vi "ConfigFunction.vi"(8 "error in (no error)":errorcluster, 11 "IviFgen in":refnum<class "IviFgen.lvclass">) -> (0 "error out":errorcluster, 3 "IviFgen out":refnum<class "IviFgen.lvclass">)   [LabVIEW 2014, in "FgenPlugins.lvlib" / "IviFgen.lvclass"]
uses:
  IviFgen.lvclass
  FgenPluginBaseClass/FgenPluginsBase.lvclass/FgenPluginsBase.ctl
  MemberClasses/StandardFunction/TypeDefs/StdWfrms.ctl
  MemberClasses/StandardFunction/TypeDefs/StdWfrm.ctl
  MemberClasses/ArbitraryFunction/TypeDefs/Arbitrary.ctl
  FgenPluginBaseClass/Accessors/Read Channels.vi
  FgenPluginBaseClass/Accessors/Read Mode (Function).vi
  FgenPluginBaseClass/Accessors/Read FunctionClass.vi
  MemberClasses/FunctionBaseClass/FunctionBase.lvclass
  MemberClasses/StandardFunction/StandardFunction.lvclass
  MemberClasses/ArbitraryFunction/ArbitraryFunction.lvclass
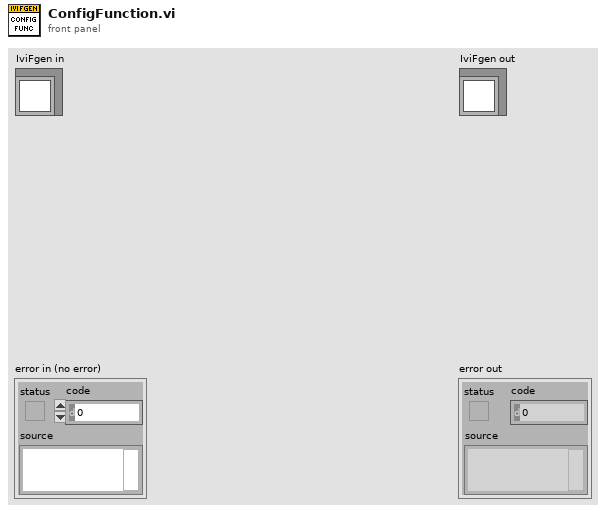
[diagram p1: front panel]
types:
  T1 = typedef "Functions.lvlib/StandardFunction.lvclass/StdWfrms.ctl" = cluster{"Count":u16, "StandardWfrm":T2[]}
  T2 = typedef "Functions.lvlib/StandardFunction.lvclass/StdWfrm.ctl" = cluster{"Amplitude":dbl, "DcOffset":dbl, "DutyCycle":dbl, "Frequency":dbl, "Phase":dbl, "Waveform":enum16{"Sine", "Square", "Triangle", "Ramp Up", "Ramp Down", "DC"}, "Handle":string}
  T3 = typedef "Functions.lvlib/ArbitraryFunction.lvclass/Arbitrary.ctl" = cluster{"Handle":string, "Size":i32, "Gain":dbl, "Offset":dbl, "Waveform":waveform(dbl)}
  T4 = typedef "FgenPlugins.lvlib/Channel.ctl" = cluster{"Name":string, "Enabled":bool, "Operation":enum16{"Continuous", "Burst"}, "Impedance (50)":dbl, "Handle":string, "Connected":bool, "Mode (Function)":enum16{"Function", "Arbitrary", "Sequence"}}
  T5 = enum16{"Sine", "Square", "Triangle", "Ramp Up", "Ramp Down", "DC"}
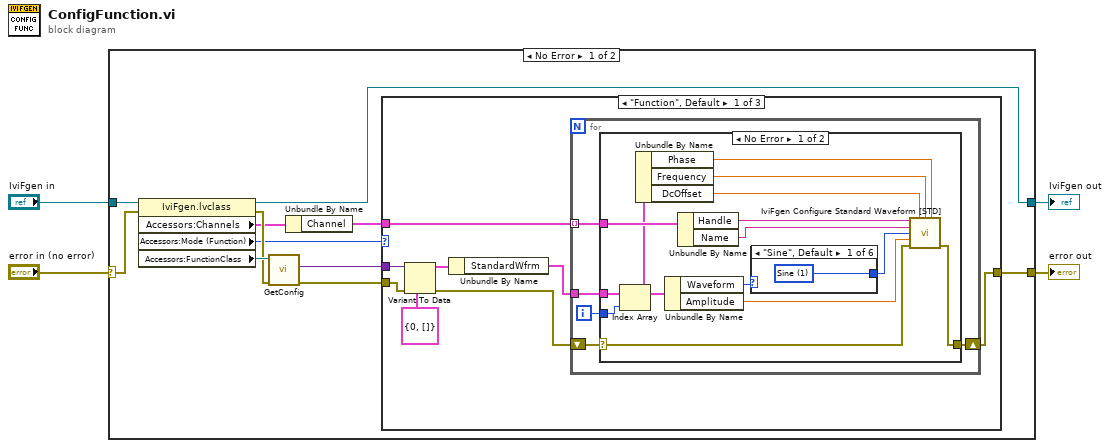
[diagram p0: block diagram]
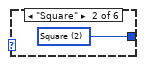
[diagram p2: hidden frame]
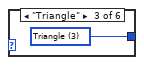
[diagram p3: hidden frame]
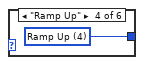
[diagram p4: hidden frame]
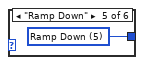
[diagram p5: hidden frame]
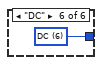
[diagram p6: hidden frame]
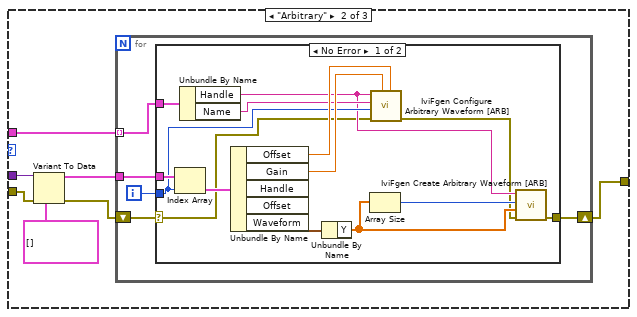
[diagram p8: hidden frame]
diagram:
  n1 = case shown="No Error" "error in (no error)" {
    selector: "error in (no error)" -> [w14 w79]
    tunnel: "IviFgen in" -> [w15 w78]
    tunnel: [w9 w79] -> w2
    tunnel: [w5 w78] -> w1
    frame No Error {
      n2 = property class="IviFgen.lvclass"(reference=w15, error in=w14) -> (reference out=w5:refnum<class "IviFgen.lvclass">, error out=w11:errorcluster, "Accessors:Channels"=w7:cluster{"Count":u16, "Channel":T4[]}, "Accessors:Mode (Function)"=w8:enum16{"Function", "Arbitrary", "Sequence"}, "Accessors:FunctionClass"=w13:refnum<class "FunctionBase.lvclass">)
      n3 = call-dynamic "GetConfig.vi"("error in (no error)"=w11, "FunctionBase in"=w13) -> ("error out"=w10:errorcluster, "Config"=w12:variant)  [unwired: 7 in, 1 out]
      n4 = Unbundle By Name(w7) -> ("Channel"=w6:T4[])
      n5 = case shown="\"Function\", Default" w8 {
        tunnel: w12 -> [w22 w56 _]
        tunnel: w10 -> [w23 w55 w77]
        tunnel: [w17 w50 w77] -> w9
        tunnel: w6 -> [w16 w53 _]
        frame "Function", Default {
          n6 = Variant To Data(error in=w23, type=T1 {"Count"=0, "StandardWfrm"=[]} ("StandardWfrms"), Variant=w22) -> (data=w20:T1, error out=w18:errorcluster)
          n7 = Unbundle By Name(w20) -> ("StandardWfrm"=w19:T2[])
          n8 = for {
            tunnel: w16 -> [w26] mode=indexing
            tunnel: w19 -> [w28]
            shift-right: [w24] -> w17
            shift-left: w18 -> [w25]
            i -> [w27]
            n9 = case shown="No Error" w25 {
              selector: w25 -> [w32 w49]
              tunnel: w28 -> [w42 _]
              tunnel: w27 -> [w41 _]
              tunnel: w26 -> [w40 _]
              tunnel: [w31 w49] -> w24
              frame No Error {
                n10 = Index Array(array=w42, index=w41) -> (element=w34:T2)
                n11 = Unbundle By Name(w34) -> ("Phase"=w35:dbl, "Frequency"=w36:dbl, "DcOffset"=w37:dbl)
                n12 = Unbundle By Name(w34) -> ("Waveform"=w30:T5, "Amplitude"=w33:dbl)
                n13 = Unbundle By Name(w40) -> ("Handle"=w39:string, "Name"=w38:string)
                n14 = case shown="\"Sine\", Default" w30 {
                  tunnel: [w43 w44 w45 w46 w47 w48] -> w29
                  frame "Sine", Default {
                    w43 = 1 items=["Sine"=1, "Square"=2, "Triangle"=3, "Ramp Up"=4, "Ramp Down"=5, "DC"=6] ("waveform (Sine)")
                  }
                  frame "Square" {
                    w44 = 2 items=["Sine"=1, "Square"=2, "Triangle"=3, "Ramp Up"=4, "Ramp Down"=5, "DC"=6] ("waveform (Sine)")
                  }
                  frame "Triangle" {
                    w45 = 3 items=["Sine"=1, "Square"=2, "Triangle"=3, "Ramp Up"=4, "Ramp Down"=5, "DC"=6] ("waveform (Sine)")
                  }
                  frame "Ramp Up" {
                    w46 = 4 items=["Sine"=1, "Square"=2, "Triangle"=3, "Ramp Up"=4, "Ramp Down"=5, "DC"=6] ("waveform (Sine)")
                  }
                  frame "Ramp Down" {
                    w47 = 5 items=["Sine"=1, "Square"=2, "Triangle"=3, "Ramp Up"=4, "Ramp Down"=5, "DC"=6] ("waveform (Sine)")
                  }
                  frame "DC" {
                    w48 = 6 items=["Sine"=1, "Square"=2, "Triangle"=3, "Ramp Up"=4, "Ramp Down"=5, "DC"=6] ("waveform (Sine)")
                  }
                }
                n15 = call <vilib>:"IviFgen Configure Standard Waveform [STD].vi"("instrument handle"=w39, "dc offset (0.00 V)"=w37, "frequency (1000.0 Hz)"=w36, "start phase (0.00 Degrees)"=w35, "channel name (\"CHANNEL1\")"=w38, "waveform (Sine)"=w29, "amplitude (1.00 V)"=w33, "error in (no error)"=w32) -> ("error out"=w31:errorcluster)  [unwired: 6 in, 1 out]
              }
              frame Error {
              }
            }
          }
        }
        frame "Arbitrary" {
          n16 = Variant To Data(error in=w55, type=T3[] [], Variant=w56) -> (data=w52:T3[], error out=w51:errorcluster)
          n17 = for {
            tunnel: w53 -> [w60] mode=indexing
            tunnel: w52 -> [w61]
            shift-right: [w58] -> w50
            shift-left: w51 -> [w57]
            i -> [w59]
            n18 = case shown="No Error" w57 {
              selector: w57 -> [w62 w76]
              tunnel: w61 -> [w75 _]
              tunnel: w60 -> [w73 _]
              tunnel: w59 -> [w69 _]
              tunnel: [w63 w76] -> w58
              frame No Error {
                n19 = Index Array(array=w75, index=w69) -> (element=w74:T3)
                n20 = Unbundle By Name(w73) -> ("Handle"=w67:string, "Name"=w70:string)
                n21 = Unbundle By Name(w74) -> ("Offset"=w72:dbl, "Gain"=w71:dbl, "Waveform"=w68:waveform(dbl))  [unwired: 2 out]
                n22 = Unbundle By Name(w68) -> ("Y"=w66:dbl[])
                n23 = Array Size(array=w66) -> (size(s)=w65:i32)
                n24 = call <vilib>:"IviFgen Configure Arbitrary Waveform [ARB].vi"("offset (0.00 V)"=w72, "gain (1.00)"=w71, "error in (no error)"=w62, "waveform handle (0)"=w69, "channel name (\"CHANNEL1\")"=w70, "instrument handle"=w67) -> ("error out"=w64:errorcluster)  [unwired: 4 in, 1 out]
                n25 = call <vilib>:"IviFgen Create Arbitrary Waveform [ARB].vi"("error in (no error)"=w64, "waveform data array (empty)"=w66, "waveform size (0)"=w65, "instrument handle"=w67) -> ("error out"=w63:errorcluster)  [unwired: 5 in, 2 out]
              }
              frame Error {
              }
            }
          }
        }
        frame "Sequence" {
          # "TBD"
        }
      }
    }
    frame Error {
    }
  }
  "error out" <- w2
  "IviFgen out" <- w1
